vi "RS232ComPort ReleaseSemaphore.vi"(8 "error in (no error)":errorcluster, 11 "RS232ComPort in":refnum<class "RS232ComPort.lvclass">) -> (0 "error out":errorcluster, 3 "RS232ComPort out":refnum<class "RS232ComPort.lvclass">)   [LabVIEW 2018, in "RS232ComPort.lvclass"]
doc: "Channel status\n -1 | Not in used so far\n 0 | For Gauge\n 1 | For 999\n100 | For 0..99\n127 | Laser"
uses:
  RS232ComPort.lvclass
  RS232ComPort.lvclass/RS232ComPort.ctl
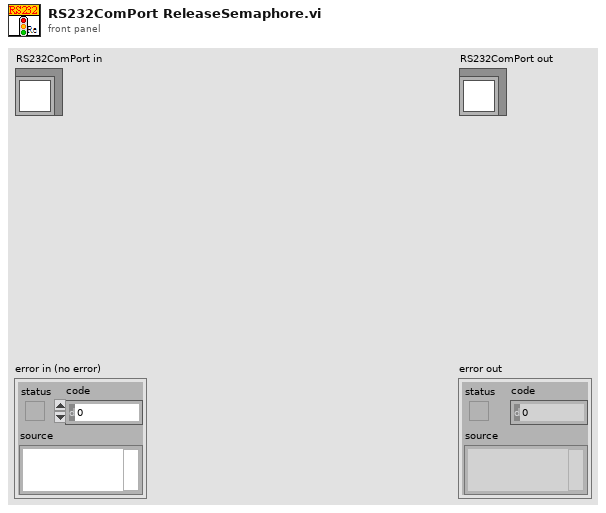
[diagram p1: front panel]
types:
  T1 = typedef "Semaphore RefNum" = refnum<k1>
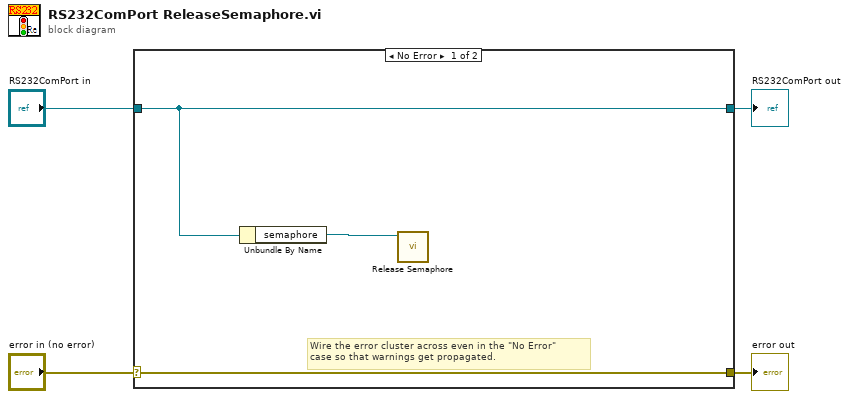
[diagram p0: block diagram]
diagram:
  n1 = case shown="No Error" "error in (no error)" {
    selector: "error in (no error)" -> [w7 w9]
    tunnel: [w7 w9] -> w3
    tunnel: [w6 w8] -> w1
    tunnel: "RS232ComPort in" -> [w6 w8]
    frame No Error {
      # "Wire the error cluster across even in the \"No Error\"\ncase so that warnings get propagated."
      n2 = Unbundle By Name(w6) -> ("semaphore"=w5:T1)
      n3 = call <vilib>:"Release Semaphore.vi"("semaphore"=w5) -> ()  [unwired: 5 in, 2 out]
    }
    frame Error {
    }
  }
  "error out" <- w3
  "RS232ComPort out" <- w1
